vi "DrawName.vi"(8 "error in (no error)":errorcluster, 11 "Highscore in":refnum<class "HighscoreDialog.lvclass">) -> (0 "error out":errorcluster, 3 "Highscore out":refnum<class "HighscoreDialog.lvclass">)   [LabVIEW 2019, in "RT_Game.lvlib" / "HighscoreDialog.lvclass"]
uses:
  HighscoreDialog.lvclass
  C:/Users/FreshBob/Dropbox/VIs/myRIO_GameConsole/RT/RT_Game/GameObject/GameObject.lvclass
  Engine/Coordinate.ctl
  GameObject/GameObject.lvclass/GameObject.ctl
  HighscoreDialog.lvclass/HighscoreDialog.ctl
  GameObject/Read position.vi
  Engine/Engine.lvclass
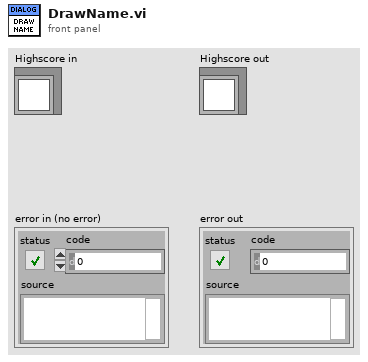
[diagram p1: front panel]
types:
  T1 = typedef "RT_Game.lvlib/Engine.lvclass/Coordinate.ctl" = cluster{"x":dbl, "y":dbl}
  T2 = typedef "RT_Game.lvlib/Game.lvclass/Coordinate.ctl" = cluster{"x":dbl, "y":dbl}
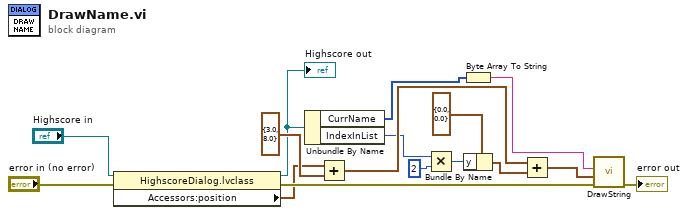
[diagram p0: block diagram]
diagram:
  n1 = property class="HighscoreDialog.lvclass"(reference="Highscore in", error in="error in (no error)") -> (reference out=w2:refnum<class "HighscoreDialog.lvclass">, error out=w4:errorcluster, "Accessors:position"=w1:T2)
  "Highscore out" <- w2
  n2 = Unbundle By Name(w2) -> ("CurrName"=w14:u8[], "IndexInList"=w8:i16)
  n3 = Add(x=w1, y=T1 {"x"=3.0, "y"=8.0}) -> (x+y=w11:T2)
  n4 = Multiply(x=w8, y=i16 2) -> (x*y=w6:i16)
  n5 = Byte Array To String(unsigned byte array=w14) -> (string=w13:string)
  n6 = Bundle By Name(cluster=T1 {"x"=0.0, "y"=0.0} ("y"), "y"=w6) -> (w9:T1)
  n7 = Add(x=w11, y=w9) -> (x+y=w5:T2)
  n8 = call "DrawString.vi"("error in (no error)"=w4, "Coordinate"=w5, "String"=w13) -> ("error out"=→"error out":errorcluster)  [unwired: 8 in]
